vi "NumberofPhases.vi"(11 "Device Properties":T1 {"Phases"."Phase Select" items=["Phase ALL", "Phase A", "Phase B", "Phase C"]}) -> (3 "error out":errorcluster, 5 "Boolean":bool)   [LabVIEW 2018, in "AcPwrPlugins.lvlib" / "ChromaAcLoad.lvclass"]
doc: "This VI checks if the number of phases is greater than three and returns a boolean true if it is."
uses:
  ChromaAcLoad.lvclass
  TypeDefs/DeviceProperties.ctl
  <vilib>/Utility/error.llb/Error Cluster From Error Code.vi
  <vilib>/ErrorRing/Error Ring.xnode
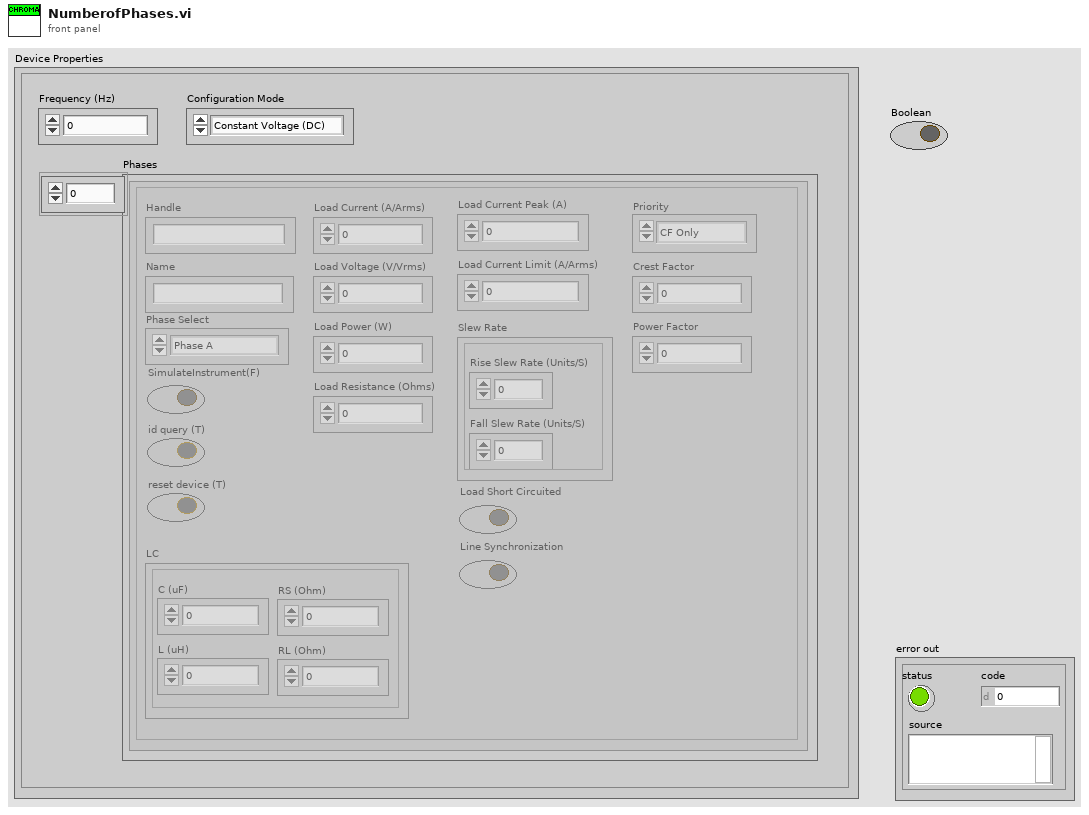
[diagram p1: front panel]
types:
  T1 = typedef "AcPwrPlugins.lvlib/ChromaAcLoad.lvclass/DeviceProperties.ctl" = cluster{"Frequency (Hz)":dbl, "Phases":cluster{"Handle":string, "Name":string, "Phase Select":i32, "SimulateInstrument(F)":bool, "id query (T)":bool, "reset device (T)":bool, "LC":cluster{"C (uF)":i32, "L (uH)":i32, "RS (Ohm)":dbl, "RL (Ohm)":dbl}, "Load Current (A/Arms)":dbl, "Load Voltage (V/Vrms)":dbl, "Load Power (W)":dbl, "Load Resistance (Ohms)":dbl, "Load Current Peak (A)":dbl, "Load Current Limit (A/Arms)":dbl, "Slew Rate":cluster{"Rise Slew Rate (Units/S)":i32, "Fall Slew Rate (Units/S)":i32}, "Load Short Circuited":bool, "Line Synchronization":bool, "Priority":enum16{"CF Only", "PF Only", "Both (CF)", "Both (PF)"}, "Crest Factor":dbl, "Power Factor":dbl, "Connected":bool, "Voltage Range (V)":dbl[], "Timing":cluster{"TimingOn":enum16{""}, "Hours":u32, "Minutes":u32, "Seconds":dbl, "CutoffVoltage":dbl}}[], "Configuration Mode":enum16{"Constant Voltage (DC)", "Constant Power (DC)", "Constant Power (AC)", "Constant Current (DC)", "Constant Current (AC)", "Constant Resistance (DC)", "Constant Resistance (AC)", "Rectified Mode (DC)", "Inrush (AC)", "RLC CP (AC)", "RLC (AC)"}}
  T2 = cluster{"Handle":string, "Name":string, "Phase Select":i32, "SimulateInstrument(F)":bool, "id query (T)":bool, "reset device (T)":bool, "LC":cluster{"C (uF)":i32, "L (uH)":i32, "RS (Ohm)":dbl, "RL (Ohm)":dbl}, "Load Current (A/Arms)":dbl, "Load Voltage (V/Vrms)":dbl, "Load Power (W)":dbl, "Load Resistance (Ohms)":dbl, "Load Current Peak (A)":dbl, "Load Current Limit (A/Arms)":dbl, "Slew Rate":cluster{"Rise Slew Rate (Units/S)":i32, "Fall Slew Rate (Units/S)":i32}, "Load Short Circuited":bool, "Line Synchronization":bool, "Priority":enum16{"CF Only", "PF Only", "Both (CF)", "Both (PF)"}, "Crest Factor":dbl, "Power Factor":dbl, "Connected":bool, "Voltage Range (V)":dbl[], "Timing":cluster{"TimingOn":enum16{""}, "Hours":u32, "Minutes":u32, "Seconds":dbl, "CutoffVoltage":dbl}}[]
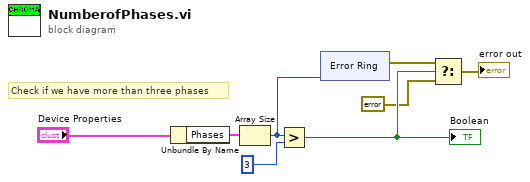
[diagram p0: block diagram]
diagram:
  # "Check if we have more than three phases"
  n1 = Unbundle By Name("Device Properties") -> ("Phases"=w7:T2)
  n2 = Array Size(array=w7) -> (size(s)=w5:i32)
  n3 = Greater?(x=w5, y=3) -> (0:w2:bool)
  "Boolean" <- w2
  n4 = xnode "Error Ring"("parameter 0"=w5) -> ("error out"=w4:errorcluster)
  n5 = Select(t=w4, s=w2, f=errorcluster {"status"=FALSE, "code"=0, "source"=""}) -> (s? t:f=→"error out":errorcluster)
